vi "Array of Waveforms.vi"(7 "amplitude 4":dbl, 8 "error in (no error)":errorcluster, 9 "amplitude 3":dbl, 10 "amplitude 2":dbl, 11 "amplitude 1":dbl) -> (0 "error out":errorcluster, 3 "waveforms":waveform(dbl)[](array[waveform]))   [LabVIEW 2023, in "Waveforms.lvlib"]
doc: "Demonstrates how to use the LabVIEW Unit Test Framework Toolkit to check VIs which contain arrays of clusters for functional correctness. The test file for this VI, Array of Waveforms.lvtest, is configured to fail."
uses:
  Waveforms.lvlib
  <vilib>/measure/NI_MABase.lvlib
panel:
  # "Overview: Demonstrates how to use the LabVIEW Unit Test Framework Toolkit to check VIs which contain arrays of clusters for functional correctness. \nRequirements: LabVIEW Full Development System, Unit Test Framework Toolkit\nInstructions:\n1.  Execute the Array of Waveforms.lvtest file for this VI. In the Project Explorer window, expand the Unit Test Files folder, right-click Array of Waveforms.lvtest, and select Run from the shortcut menu.\n2.  View the test results in the Unit Test Framework Results window, which shows that this test fails."
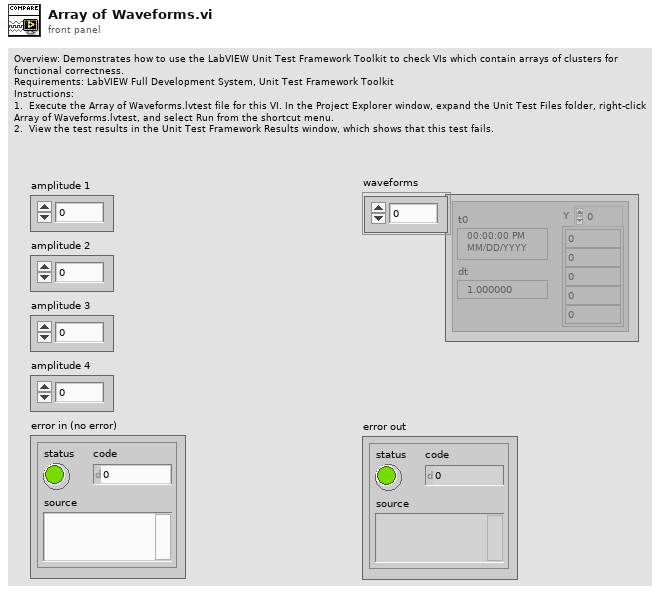
[diagram p1: front panel]
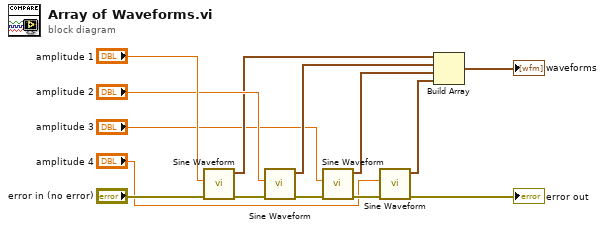
[diagram p0: block diagram]
diagram:
  n1 = call <vilib>:"Sine Waveform.vi"("error in (no error)"="error in (no error)", "amplitude"="amplitude 1") -> ("error out"=w13:errorcluster, "signal out"=w4:waveform(dbl))  [unwired: 5 in, 3 out]
  n2 = call <vilib>:"Sine Waveform.vi"("error in (no error)"=w13, "amplitude"="amplitude 2") -> ("error out"=w12:errorcluster, "signal out"=w5:waveform(dbl))  [unwired: 5 in, 3 out]
  n3 = call <vilib>:"Sine Waveform.vi"("error in (no error)"=w12, "amplitude"="amplitude 3") -> ("error out"=w11:errorcluster, "signal out"=w6:waveform(dbl))  [unwired: 5 in, 3 out]
  n4 = call <vilib>:"Sine Waveform.vi"("error in (no error)"=w11, "amplitude"="amplitude 4") -> ("error out"=→"error out":errorcluster, "signal out"=w7:waveform(dbl))  [unwired: 5 in, 3 out]
  n5 = Build Array(w4, w5, w6, w7) -> (→"waveforms":waveform(dbl)[])
